vi "References.vi"(9 "Cluster":T1, 10 "VI Refnum":refnum<vi>, 11 "TS.SequenceContext":refnum<k7>) -> ()   [LabVIEW 2013]
panel:
  in  "stop":bool
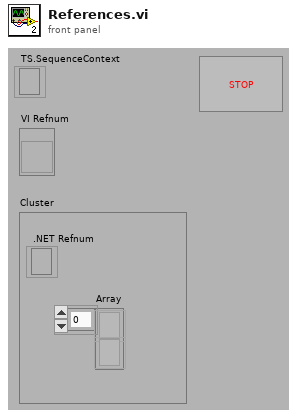
[diagram p1: front panel]
types:
  T1 = cluster{".NET Refnum":refnum<k24>, "Array":refnum<k7>[]}
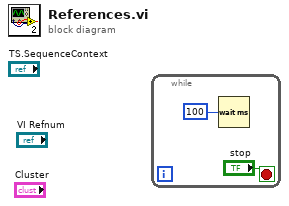
[diagram p0: block diagram]
diagram:
  n1 = while {
    stop <- "stop" stop-if-true
    n2 = Wait (ms)(milliseconds to wait=u32 100) -> ()  [unwired: 1 out]
  }
